vi "GE 5565PIORC.DMA.Scatter-Gather.vi"(10 "number of blocks (10)":i32=10, 11 "count per block (1000)":u32=1000) -> (0 "error out":errorcluster, 3 "pass?":bool)   [LabVIEW 2017]
uses:
  Source/GE 5565PIORC.lvclass/GE 5565PIORC.ctl
  Source/Methods/GE 5565PIORC.DMA.Block.Write (DBL).vi
  Source/Methods/GE 5565PIORC.DMA.Create Transfer (Scatter-Gather).vi
  Source/Methods/GE 5565PIORC.DMA.Block.Read (DBL).vi
  Source/Properties/Registers/GE 5565PIORC.Registers.DMACSR0.Channel 0 Enable.Set.vi
  Source/Properties/GE 5565PIORC.Read VISA MEMACC.vi
  Source/Methods/GE 5565PIORC.DMA.Size.vi
  Source/Methods/GE 5565PIORC.DMA.Configure.vi
  Source/Methods/GE 5565PIORC.PXI Interrupts.Discard Events.vi
  Source/Methods/GE 5565PIORC.DMA.Start.vi
  Source/Methods/GE 5565PIORC.DMA.Wait for Done.vi
  Source/Properties/Registers/GE 5565PIORC.Registers.Local Configuration.Read.vi
  Source/Properties/Registers/GE 5565PIORC.Registers.Local Configuration.Read (U8).vi
  Source/Properties/Registers/GE 5565PIORC.Registers.Local Configuration.Write.vi
  Source/Properties/Registers/GE 5565PIORC.Registers.Local Configuration.Write (U8).vi
  Source/Methods/GE 5565PIORC.Bit Manipulation.Set Bit.vi
  Source/Methods/GE 5565PIORC.Bit Manipulation.Set Bit (U8).vi
  Source/Properties/Registers/GE 5565PIORC.Registers.DMADPR0.Direction of Transfer.Set.vi
  Source/Properties/Registers/GE 5565PIORC.Registers.DMASIZ0.DMA Transfer Size.Set.vi
  Source/Properties/Registers/GE 5565PIORC.Registers.DMALADR0.Local Address Register.Set.vi
  Source/Properties/Registers/GE 5565PIORC.Registers.DMAMODE0.Scatter-Gather Mode.Set.vi
  Source/Properties/Registers/GE 5565PIORC.Registers.DMAPADR0.PCI Address Register.Set.vi
  Source/Methods/GE 5565PIORC.DMA.Scatter-Gather.Link Block Descriptors.vi
  Source/Methods/GE 5565PIORC.DMA.Scatter-Gather.Commit Linked Block Descriptors.vi
  Source/Properties/Registers/GE 5565PIORC.Registers.DMADPR0.Channel 0 First Descriptor Address.Set.vi
  Source/Methods/GE 5565PIORC.DMA.Get Transfer Components.vi
  Source/Methods/GE 5565PIORC.DMA.Get Transfer Components (Scatter-Gather).vi
  <vilib>/Utility/error.llb/Clear Errors.vi
  Source/Properties/Registers/GE 5565PIORC.Registers.DMACSR0.Channel 0 Start.Set.vi
  Source/Properties/Registers/GE 5565PIORC.Registers.DMACSR0.Channel 0 Clear Interrupt.Set.vi
  Source/Methods/GE 5565PIORC.DMA.Poll for Done Signal.vi
  Source/Methods/GE 5565PIORC.PXI Interrupts.Wait for Event.vi
  Source/Methods/GE 5565PIORC.Registers.Read.vi
  Source/Methods/GE 5565PIORC.Registers.Read (U8).vi
  Source/Methods/GE 5565PIORC.Registers.Write.vi
  Source/Methods/GE 5565PIORC.Registers.Write (U8).vi
  Source/Properties/Registers/GE 5565PIORC.Registers.Local Configuration.Read (U32).vi
  Source/Properties/Registers/GE 5565PIORC.Registers.Local Configuration.Write (U32).vi
  Source/Methods/GE 5565PIORC.Bit Manipulation.Set Bit (U32).vi
  Source/Methods/GE 5565PIORC.DMA.Scatter-Gather.Set Descriptor Params.vi
  Source/Methods/GE 5565PIORC.DMA.Is Done.vi
  Source/Methods/GE 5565PIORC.Registers.Read (U32).vi
  Source/Methods/GE 5565PIORC.Registers.Write (U32).vi
  Source/Properties/Registers/GE 5565PIORC.Registers.DMACSR0.Channel 0 Inactive.Get.vi
  Source/Methods/GE 5565PIORC.Bit Manipulation.Get Bit.vi
  Source/Methods/GE 5565PIORC.Bit Manipulation.Get Bit (U8).vi
  Source/Methods/GE 5565PIORC.Round Up to Nearest 8.vi
  Source/Methods/GE 5565PIORC.Round Up to Nearest 16.vi
  Source/GE 5565PIORC.lvclass
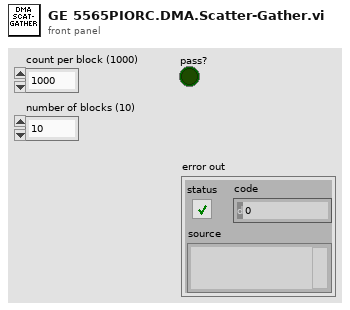
[diagram p1: front panel]
types:
  T1 = typedef "GE 5565PIORC.lvclass/GE 5565PIORC.Typedef.DMA Block Descriptor.ctl" = cluster{"descriptor ptr (VISA)":u32, "descriptor ptr (RFM)":u32, "descriptor size":u32, "descriptor params":T2}
  T2 = typedef "GE 5565PIORC.lvclass/GE 5565PIORC.Typedef.DMA Block Descriptor Params.ctl" = cluster{"data ptr (lower)":u32, "data ptr (upper)":u32, "data size":u32, "next descriptor ptr":u32}
  T3 = typedef "GE 5565PIORC.lvclass/GE 5565PIORC.Typedef.DMA Transfer Spec.ctl" = cluster{"RFM offset":u32, "Block Descriptors":T1[]}
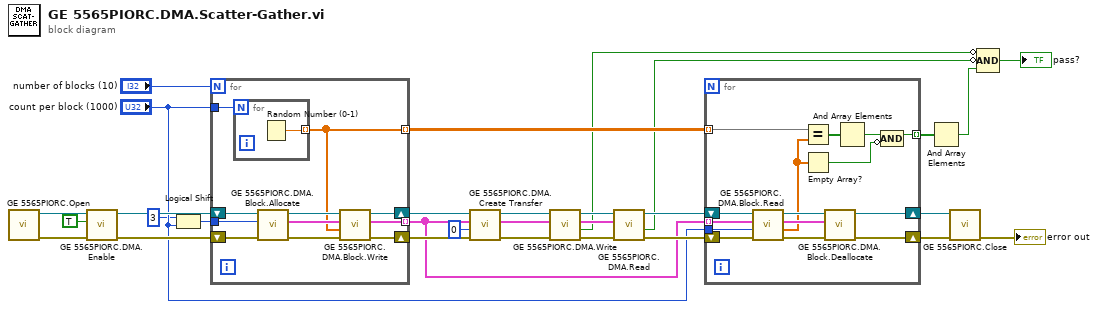
[diagram p0: block diagram]
diagram:
  n1 = call "GE 5565PIORC.Open.vi"() -> ("error out"=w26:errorcluster, "GE 5565PIORC"=w27:refnum<class "GE 5565PIORC.lvclass">)  [unwired: 10 in]
  n2 = call "GE 5565PIORC.DMA.Enable.vi"("error in (no error)"=w26, "enable (T)"=TRUE ("Enable DMA"), "GE 5565PIORC in"=w27) -> ("error out"=w28:errorcluster, "GE 5565PIORC out"=w29:refnum<class "GE 5565PIORC.lvclass">)  [unwired: 7 in]
  n3 = Logical Shift(y=i16 3, x="count per block (1000)") -> (x << y=w23:u32)
  n4 = for {
    N: "number of blocks (10)" -> [_]
    tunnel: [w34] -> w18 mode=indexing
    tunnel: "count per block (1000)" -> [w39]
    shift-right: [w33] -> w22
    shift-left: w29 -> [w41]
    shift-right: [w32] -> w21
    shift-left: w28 -> [w40]
    tunnel: w23 -> [w38]
    tunnel: [w31] -> w17 mode=indexing
    n5 = for {
      N: w39 -> [_]
      tunnel: [w42] -> w34 mode=indexing
      n6 = Random Number (0-1)() -> (number: 0 to 1=w42:dbl)
    }
    n7 = call "GE 5565PIORC.DMA.Block.Allocate.vi"("error in (no error)"=w40, "size in bytes"=w38, "GE 5565PIORC in"=w41) -> ("error out"=w36:errorcluster, "Block Descriptor"=w35:T1, "GE 5565PIORC out"=w37:refnum<class "GE 5565PIORC.lvclass">)  [unwired: 6 in]
    n8 = call-poly "GE 5565PIORC.DMA.Block.Write.vi"("error in (no error)"=w36, "data"=w34, "Block Descriptor in"=w35, "GE 5565PIORC in"=w37) -> ("error out"=w32:errorcluster, "Block Descriptor out"=w31:T1, "GE 5565PIORC out"=w33:refnum<class "GE 5565PIORC.lvclass">)  [unwired: 4 in, 1 out]
  }
  n9 = call-poly "GE 5565PIORC.DMA.Create Transfer.vi"("error in (no error)"=w21, "RFM offset"=u32 0, "Block Descriptors"=w17, "GE 5565PIORC in"=w22) -> ("error out"=w5:errorcluster, "DMA Transfer Spec"=w6:T3, "GE 5565PIORC out"=w7:refnum<class "GE 5565PIORC.lvclass">)  [unwired: 4 in, 1 out]
  n10 = call "GE 5565PIORC.DMA.Write.vi"("error in (no error)"=w5, "DMA Transfer Spec"=w6, "GE 5565PIORC in"=w7) -> ("error out"=w2:errorcluster, "timed out?"=w1:bool, "DMA Transfer Spec dup"=w3:T3, "GE 5565PIORC out"=w4:refnum<class "GE 5565PIORC.lvclass">)  [unwired: 5 in]
  n11 = call "GE 5565PIORC.DMA.Read.vi"("error in (no error)"=w2, "DMA Transfer Spec"=w3, "GE 5565PIORC in"=w4) -> ("error out"=w19:errorcluster, "timed out?"=w11:bool, "GE 5565PIORC out"=w20:refnum<class "GE 5565PIORC.lvclass">)  [unwired: 5 in, 1 out]
  n12 = for {
    shift-right: [w49] -> w13
    shift-left: w20 -> [w56]
    shift-right: [w48] -> w12
    shift-left: w19 -> [w55]
    tunnel: w18 -> [w47] mode=indexing
    tunnel: w17 -> [w57] mode=indexing
    tunnel: "count per block (1000)" -> [w54]
    tunnel: [w43] -> w14 mode=indexing
    n13 = call-poly "GE 5565PIORC.DMA.Block.Read.vi"("error in (no error)"=w55, "count"=w54, "Block Descriptor in"=w57, "GE 5565PIORC in"=w56) -> ("error out"=w51:errorcluster, "data out"=w46:dbl[], "Block Descriptor out"=w50:T1, "GE 5565PIORC out"=w52:refnum<class "GE 5565PIORC.lvclass">)  [unwired: 4 in]
    n14 = Equal?(x=w47, y=w46) -> (x = y?=w53:bool[])
    n15 = Empty Array?(array=w46) -> (empty?=w45:bool)
    n16 = call "GE 5565PIORC.DMA.Block.Deallocate.vi"("error in (no error)"=w51, "Block Descriptor"=w50, "GE 5565PIORC in"=w52) -> ("error out"=w48:errorcluster, "GE 5565PIORC out"=w49:refnum<class "GE 5565PIORC.lvclass">)  [unwired: 7 in]
    n17 = And Array Elements(Boolean array=w53) -> (logical AND=w44:bool)
    n18 = Compound Arithmetic op=AND(w44, invert w45) -> (w43:bool)
  }
  n19 = And Array Elements(Boolean array=w14) -> (logical AND=w8:bool)
  n20 = call "GE 5565PIORC.Close.vi"("error in (no error)"=w12, "GE 5565PIORC"=w13) -> ("error out"=→"error out":errorcluster)  [unwired: 9 in]
  n21 = Compound Arithmetic op=AND(invert w1, invert w11, w8) -> (→"pass?":bool)
